vi "Create Transfer Group.vi"(4 "FIFO options":T1, 7 "id (0)":i32, 8 "error in":errorcluster, 9 "thread index":i32, 10 "buffers":refnum<class "Buffers.lvclass">, 11 "group configuration":refnum<class "Group Configuration.lvclass">) -> (0 "error out":errorcluster, 3 "transfer group out":refnum<class "Transfer Group.lvclass">)   [LabVIEW 2021, in "DSF Core.lvlib" / "Transfer Group.lvclass"]
doc: "Create transfer group object."
uses:
  Transfer Group.lvclass
  Buffers/Buffers.lvclass
  Typedefs/DSF FIFO Options.ctl
  Configuration/Core/Group/Group Configuration.lvclass
  Buffers/Buffers.lvclass/Buffers.ctl
  <vilib>/NI/Memory Manager/Classes/Pointer/Pointer.lvclass/Pointer.ctl
  Buffer/Buffer.lvclass/Buffer.ctl
  Transfer/Transfer.lvclass/Transfer.ctl
  Timing/Timing.lvclass/Timing.ctl
  Transfer Group.lvclass/Transfer Group.ctl
  Performance/Performance.lvclass/Performance.ctl
  Transfer/Create Transfer.vi
  Buffer/Subset Buffer.vi
  <vilib>/Utility/error.llb/Clear Errors.vi
  Buffer/Set Buffer Size.vi
  Buffers/Create.vi
  Create Return FIFO.vi
  Performance/Create.vi
  <vilib>/NI/Memory Manager/Classes/Pointer/Subset.vi
  Buffer/Set Buffer Offset.vi
  <vilib>/NI/Memory Manager/Classes/Pointer/Set Size.vi
  Timing Status/Create.vi
  Timing Status/Write Timing Status.vi
  <vilib>/NI/Memory Manager/Classes/Pointer/Get Address.vi
  <vilib>/NI/Memory Manager/Classes/Pointer/Encapsulate.vi
  <vilib>/NI/Memory Manager/Classes/Pointer/Check Null Pointer.vi
  <vilib>/NI/Memory Manager/Classes/Pointer/Check Length.vi
  <vilib>/NI/Memory Manager/Classes/Pointer/Allocate.vi
  Timing Status/Timing Status Size.vi
  <vilib>/NI/Memory Manager/Classes/Pointer/Check Size.vi
  <vilib>/NI/Memory Manager/Classes/Pointer/Set Address.vi
  <vilib>/NI/Memory Manager/Classes/Pointer/Set Internal.vi
  <vilib>/NI/Memory Manager/Classes/Pointer/Errors.vi
  <vilib>/NI/Memory Manager/Classes/Pointer/Null Pointer.vi
  <vilib>/NI/Memory Manager/Classes/Pointer/Is Null.vi
  <vilib>/NI/Memory Manager/Classes/Pointer/Get Size.vi
  <vilib>/NI/Memory Manager/Classes/Pointer/Check Bounds (Pointer).vi
  <vilib>/NI/Memory Manager/Classes/Pointer/Out of Bounds.vi
  <vilib>/NI/Memory Manager/Classes/Pointer/Create Error.vi
  <vilib>/NI/Memory Manager/VIs/Write String to Source.vi
  <vilib>/NI/Memory Manager/Classes/Pointer/Write Pointer Size to Error.vi
  <vilib>/NI/Memory Manager/VIs/Write Numeric to Source.vi
  <vilib>/NI/Memory Manager/VIs/Write Numeric Scalar to Source (Base10 U64).vi
  <vilib>/NI/Memory Manager/VIs/New Error Cluster.vi
  <vilib>/NI/Memory Manager/VIs/New Error Cluster (512B).vi
  <vilib>/NI/Memory Manager/VIs/Set Error Status.vi
  <vilib>/NI/Memory Manager/VIs/Set Error Code.vi
  <vilib>/NI/Memory Manager/VIs/Set Error Source.vi
  <vilib>/NI/Memory Manager/Constants/Constants.vi
  <vilib>/NI/Memory Manager/Constants/Library Name.vi
  <vilib>/NI/Memory Manager/Classes/Pointer/Pointer Error Info.vi
  <vilib>/NI/Memory Manager/Constants/Pointer Class Name.vi
  Buffer/Buffer.lvclass
  C:/Program Files/National Instruments/LabVIEW 2021/vi.lib/NI/Memory Manager/Classes/Pointer/Pointer.lvclass
  Timing Status/Timing Status Pointer.lvclass
  Configuration/Core/Transfer/Get Name.vi
  Transfer/Transfer.lvclass
  Performance/Performance.lvclass
  Configuration/Core/Transfer/Transfer Configuration.lvclass
  Timing/Timing.lvclass
  Framework/Framework.lvclass
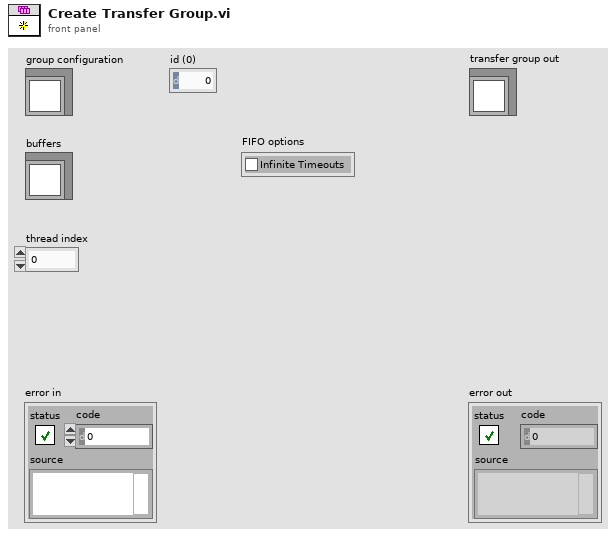
[diagram p1: front panel]
types:
  T1 = typedef "DSF Core.lvlib/Framework.lvclass/DSF FIFO Options.ctl" = cluster{"Infinite Timeouts":bool}
  T2 = typedef "DSF Core.lvlib/Group Configuration.lvclass/Core Group Configuration.ctl" = cluster{"name":string, "direction":T3, "cycle timing":T4, "timeout behavior":T5, "enable conversion":bool}
  T3 = typedef "DSF Core.lvlib/DSF Direction.ctl" = enum8{"Tx", "Rx"}
  T4 = typedef "DSF Core.lvlib/DSF Timing Info.ctl" = cluster{"priority":u64, "decimation":u64, "offset":u64}
  T5 = typedef "DSF Core.lvlib/DSF Timeout Behavior.ctl" = enum8{"Increment Late Count", "Throw Error"}
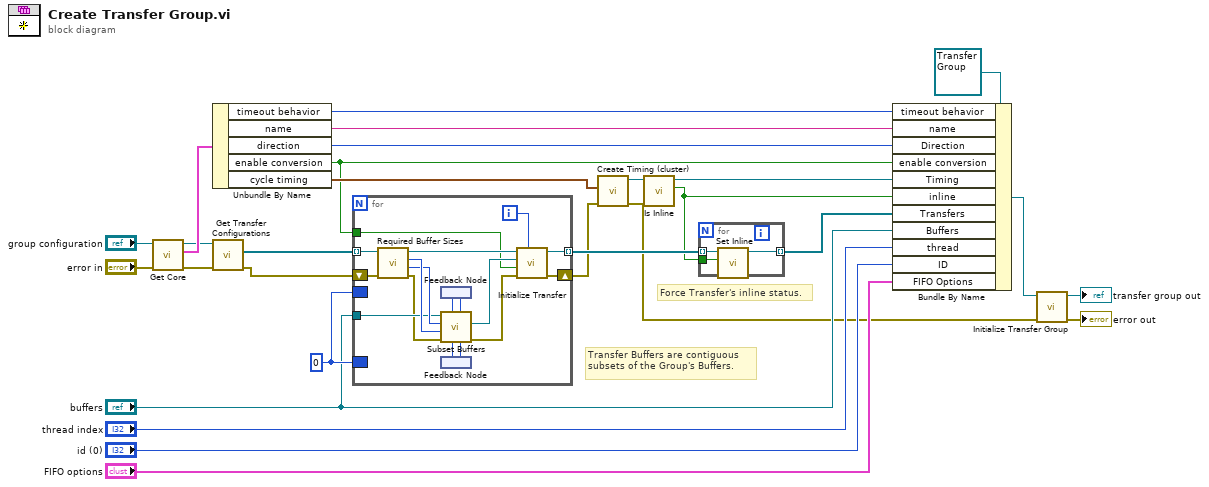
[diagram p0: block diagram]
diagram:
  w15 = u64 0 ("inline buffer size")
  # "Transfer Buffers are contiguous subsets of the Group's Buffers."
  # "Force Transfer's inline status."
  n1 = call "Get Core.vi"("error in (no error)"="error in", "Group Configuration in"="group configuration") -> ("error out"=w5:errorcluster, "core"=w14:T2, "Group Configuration out"=w4:refnum<class "Group Configuration.lvclass">)  [unwired: 7 in]
  n2 = Unbundle By Name(w14) -> ("timeout behavior"=w23:T5, "name"=w24:string, "direction"=w25:T3, "enable conversion"=w3:bool, "cycle timing"=w26:T4)
  n3 = call "Get Transfer Configurations.vi"("error in (no error)"=w5, "Group Configuration in"=w4) -> ("error out"=w2:errorcluster, "Transfer Configurations"=w9:refnum<class "Transfer Configuration.lvclass">[])  [unwired: 7 in, 1 out]
  n4 = for {
    tunnel: [w45] -> w22 mode=indexing
    border: w15 -> [_]
    border: w15 -> [_]
    tunnel: w9 -> [w37] mode=indexing
    tunnel: "buffers" -> [w34]
    tunnel: w3 -> [w32]
    shift-right: [w29] -> w1
    shift-left: w2 -> [w31]
    i -> [w44]
    n5 = call-dynamic "Required Buffer Sizes.vi"("error in (no error)"=w31, "Transfer Configuration in"=w37) -> ("error out"=w30:errorcluster, "string size"=w35:u64, "engine size"=w36:u64, "Transfer Configuration out"=w33:refnum<class "Transfer Configuration.lvclass">)  [unwired: 6 in]
    n6 = feedback #1() -> (w39:u64)
    n7 = feedback #2() -> (w38:u64)
    n8 = call "Subset Buffers.vi"("engine buffer offset"=w38, "string buffer offset"=w39, "error in (no error)"=w30, "engine buffer size"=w36, "string buffer size"=w35, "Buffers in"=w34) -> ("error out"=w41:errorcluster, "subset Buffers"=w40:refnum<class "Buffers.lvclass">, "engine buffer offset +size"=w43:u64, "string buffer offset + size"=w42:u64)  [unwired: 1 in, 1 out]
    n9 = feedback-in #1(w42) -> ()
    n10 = feedback-in #2(w43) -> ()
    n11 = call "Initialize Transfer.vi"("id"=w44, "error in (no error)"=w41, "convert (F)"=w32, "Buffers"=w40, "Transfer Configuration"=w33) -> ("error out"=w29:errorcluster, "Transfer out"=w45:refnum<class "Transfer.lvclass">)  [unwired: 5 in]
  }
  n12 = call "Create Timing (cluster).vi"("error in (no error)"=w1, "cycle timing"=w26) -> ("error out"=w8:errorcluster, "Timing"=w27:refnum<class "Timing.lvclass">)  [unwired: 8 in]
  n13 = call "Is Inline.vi"("Timing in"=w27) -> ("inline?"=w19:bool, "Timing out"=w21:refnum<class "Timing.lvclass">)  [unwired: 9 in]
  n14 = for {
    tunnel: w22 -> [w48] mode=indexing
    tunnel: w19 -> [w47]
    tunnel: [w46] -> w11 mode=indexing
    n15 = call "Set Inline.vi"("inline"=w47, "Transfer in"=w48) -> ("Transfer out"=w46:refnum<class "Transfer.lvclass">)  [unwired: 9 in]
  }
  n16 = Bundle By Name(cluster=refnum<class "Transfer Group.lvclass"> refnum ("Transfer Group type"), "timeout behavior"=w23, "name"=w24, "Direction"=w25, "enable conversion"=w3, "Timing"=w21, "inline"=w19, "Transfers"=w11, "Buffers"="buffers", "thread"="thread index", "ID"="id (0)", "FIFO Options"="FIFO options") -> (w18:refnum<class "Transfer Group.lvclass">)
  n17 = call "Initialize Transfer Group.vi"("error in (no error)"=w8, "Transfer Group in"=w18) -> ("error out"=→"error out":errorcluster, "Transfer Group out"=→"transfer group out":refnum<class "Transfer Group.lvclass">)  [unwired: 8 in]
